vi "subAxopatch_GetGain.vi"(11 "Patch AI lines 2-Gain":tag="Dev1/ai0") -> (3 "Gain (pA/V)":dbl=1000.0)   [LabVIEW 2015]
panel:
  out "AI signal (V)":dbl format="%0.2f"
  out "V_m (mV/mV)":dbl=1000.0
  out "I (mV/pA)":dbl=1000.0
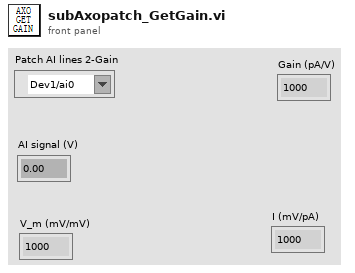
[diagram p1: front panel]
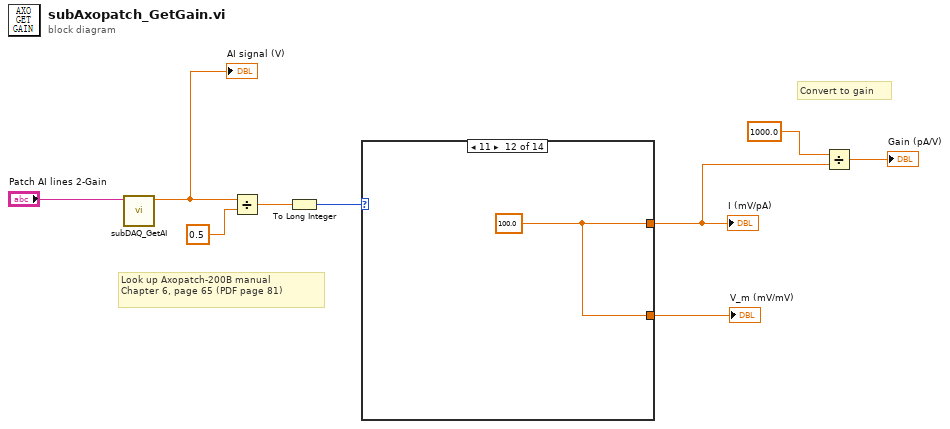
[diagram p0: block diagram]
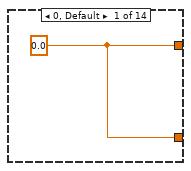
[diagram p2: hidden frame]
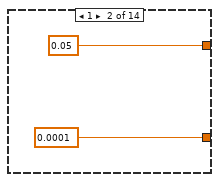
[diagram p3: hidden frame]
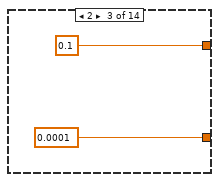
[diagram p4: hidden frame]
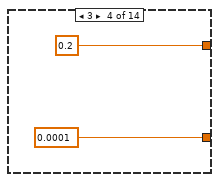
[diagram p5: hidden frame]
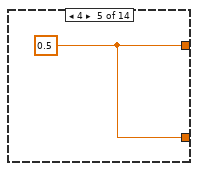
[diagram p6: hidden frame]
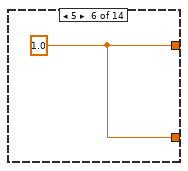
[diagram p7: hidden frame]
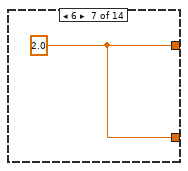
[diagram p8: hidden frame]
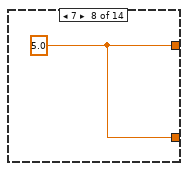
[diagram p9: hidden frame]
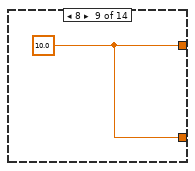
[diagram p10: hidden frame]
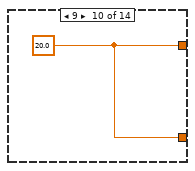
[diagram p11: hidden frame]
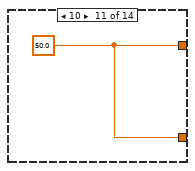
[diagram p12: hidden frame]
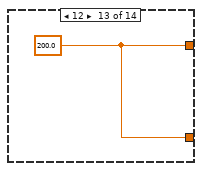
[diagram p13: hidden frame]
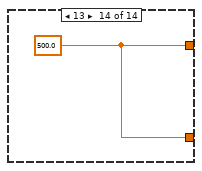
[diagram p14: hidden frame]
diagram:
  # "Convert to gain"
  # "Look up Axopatch-200B manual\nChapter 6, page 65 (PDF page 81)"
  n1 = call "subDAQ_GetAI.vi"("AI line"="Patch AI lines 2-Gain") -> ("AI signal (V)"=w8:dbl)  [unwired: 9 in, 1 out]
  "AI signal (V)" <- w8
  n2 = Divide(x=w8, y=0.5) -> (x/y=w6:dbl)
  n3 = To Long Integer(number=w6) -> (32bit integer=w5:i32)
  n4 = case shown="11" w5 {
    tunnel: [w10 0.0001 ("I (mV/pA)") 0.0001 ("I (mV/pA)") 0.0001 ("I (mV/pA)") w17 w18 w19 w20 w21 w22 w23 w24 w25 w26] -> w4
    tunnel: [w10 0.05 ("I (mV/pA)") 0.1 ("I (mV/pA)") 0.2 ("I (mV/pA)") w17 w18 w19 w20 w21 w22 w23 w24 w25 w26] -> w3
    frame 0, Default {
      w10 = 0.0 ("I (mV/pA)")
    }
    frame 1 {
    }
    frame 2 {
    }
    frame 3 {
    }
    frame 4 {
      w17 = 0.5 ("I (mV/pA)")
    }
    frame 5 {
      w18 = 1.0 ("I (mV/pA)")
    }
    frame 6 {
      w19 = 2.0 ("I (mV/pA)")
    }
    frame 7 {
      w20 = 5.0 ("I (mV/pA)")
    }
    frame 8 {
      w21 = 10.0 ("I (mV/pA)")
    }
    frame 9 {
      w22 = 20.0 ("I (mV/pA)")
    }
    frame 10 {
      w23 = 50.0 ("I (mV/pA)")
    }
    frame 11 {
      w24 = 100.0 ("I (mV/pA)")
    }
    frame 12 {
      w25 = 200.0 ("I (mV/pA)")
    }
    frame 13 {
      w26 = 500.0 ("I (mV/pA)")
    }
  }
  "I (mV/pA)" <- w3
  "V_m (mV/mV)" <- w4
  n5 = Divide(x=1000.0, y=w3) -> (x/y=→"Gain (pA/V)":dbl)
